vi "Stop Core.vi"(10 "final error code":i32, 11 "App in":refnum<class "App.lvclass">) -> (3 "App out":refnum<class "App.lvclass">)   [LabVIEW 2016, in "App.lvlib" / "App.lvclass"]
doc: "(<B>Filename</B>: Actor Framework.lvlib:Actor.lvclass:Stop Core.vi)\n\nDefines what the actor does before it stops. Use the <B>final error code</B> input to determine whether the actor shut down in response to an error.\n\nBy default, this method does nothing. A descendant class may override it to define behavior, such as shutting down any processes the actor initiated in its override of the Actor Core method."
uses:
  App.lvclass
  App.lvclass/App.ctl
  <vilib>/ActorFramework/Actor/Actor.lvclass
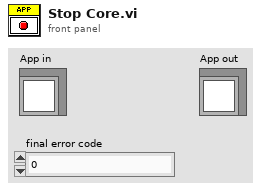
[diagram p1: front panel]
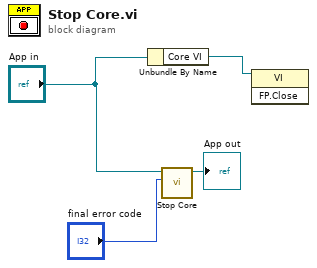
[diagram p0: block diagram]
diagram:
  n1 = Unbundle By Name("App in") -> ("Core VI"=w1:refnum<vi>)
  n2 = call-parent "Stop Core.vi"("final error code"="final error code", "Actor in"="App in") -> ("Actor out"=→"App out":refnum<class "App.lvclass">)  [unwired: 9 in]
  n3 = invoke class="VI" method="FP.Close"(reference=w1) -> ()  [unwired: 2 in, 3 out]
